vi "GetHW_ID.vi"(8 "error in (no error)":errorcluster, 11 "AdaFruit-Seesaw in":refnum<class "AdaFruit-Seesaw.lvclass">) -> (0 "error out":errorcluster, 2 "HW_ID":string, 3 "AdaFruit-Seesaw out":refnum<class "AdaFruit-Seesaw.lvclass">)   [LabVIEW 2020, in "CTI-Peripheral.lvlib" / "AdaFruit-Seesaw.lvclass"]
uses:
  AdaFruit-Seesaw.lvclass
  Private/SeeSawBaseAddresses.ctl
  Private/SeeSawSTATUSFunctions.ctl
  AdaFruit-Seesaw.lvclass/AdaFruit-Seesaw.ctl
  CTI/I2C Connection/I2C Connection.lvclass/I2C Connection.ctl
  CTI/Session/I2C Write Data.vi
  CTI/Session/I2C Read Data.vi
  CTI/I2C Connection/I2C Connection.lvclass
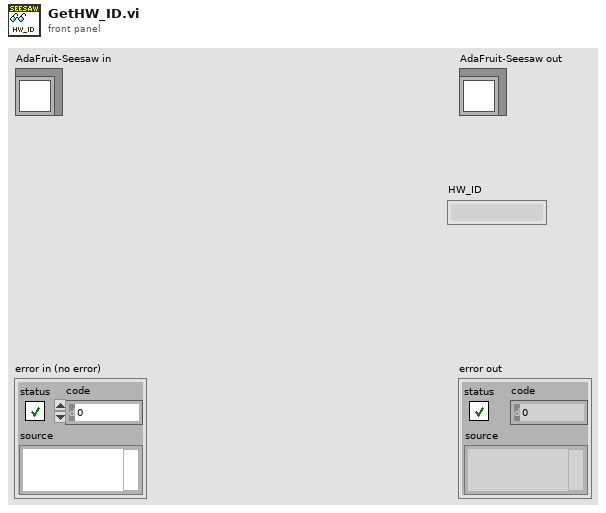
[diagram p1: front panel]
types:
  T1 = typedef "CTI-Peripheral.lvlib/AdaFruit-Seesaw.lvclass/SeeSawSTATUSFunctions.ctl" = u8
  T2 = typedef "CTI-Peripheral.lvlib/AdaFruit-Seesaw.lvclass/SeeSawBaseAddresses.ctl" = u8
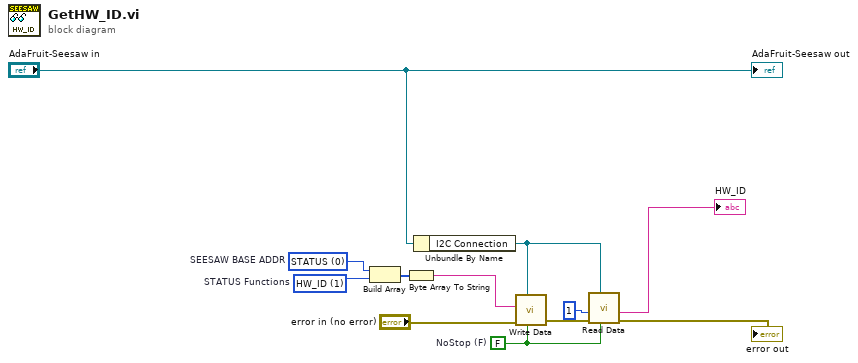
[diagram p0: block diagram]
diagram:
  w1 = T1 1 items=["HW_ID"=1, "VERSION"=2, "OPTIONS"=3, "TEMP"=4, "SWRST"=7]  # STATUS Functions
  w7 = FALSE  # NoStop (F)
  w12 = T2 0 items=["STATUS"=0, "GPIO"=1, "SERCOM0"=2, "TIMER"=8, "ADC"=9, "DAC"=10, "INTERUPT"=11, "DAP"=12, "EEPROM"=13, "NEOPIXEL"=14, "TOUCH"=15, "KEYPAD"=16, "ENCODER"=17, "SPECTRUM"=18]  # SEESAW BASE ADDR
  n1 = Build Array(w12, w1) -> (w11:T1[])
  n2 = Byte Array To String(unsigned byte array=w11) -> (string=w6:string)
  n3 = Unbundle By Name("AdaFruit-Seesaw in") -> ("I2C Connection"=w8:refnum<class "I2C Connection.lvclass">)
  n4 = call "Write Data.vi"("NoStop (F)"=w7, "I2C Connection"=w8, "error in (no error)"="error in (no error)", "Data"=w6) -> ("error out"=w10:errorcluster)  [unwired: 7 in]
  n5 = call "Read Data.vi"("NoStop (F)"=w7, "I2C Connection"=w8, "error in (no error)"=w10, "Len"=u8 1 ("Read Len")) -> ("error out"=→"error out":errorcluster, "Data"=→"HW_ID":string)  [unwired: 6 in]
  "AdaFruit-Seesaw out" <- "AdaFruit-Seesaw in"
